vi "Joystick Outputs.vi"(0 "JoystickDevRef":T1) -> (1 "Buttons":T4, 2 "Axis":T3, 3 "POV":cluster{"POV":i16})   [LabVIEW 2020]
uses:
  <vilib>/Rock Robotics/WPI/Joystick/WPI_JoystickDevRef.ctl
  <vilib>/Rock Robotics/WPI/Joystick/WPI_JoystickDeviceEnum.ctl
panel:
  out "POV BL":bool
  out "POV BR":bool
  out "POV TR":bool
  out "POV TR":bool
  out "POV B":bool
  out "POV T":bool
  out "POV L":bool
  out "POV R":bool
  out "POV C":bool
  out "\"x' 13":bool
  out "\"x' 12":bool
  out "\"x' 11":bool
  out "\"x' 10":bool
  out "\"x' 9":bool
  out "\"x' 8":bool
  out "\"x' 7":bool
  out "\"x' 2":bool
  out "\"x' 6":bool
  out "\"x' 4":bool
  out "\"x' 3":bool
  out "\"x' 2":bool
  out "\"x'":bool
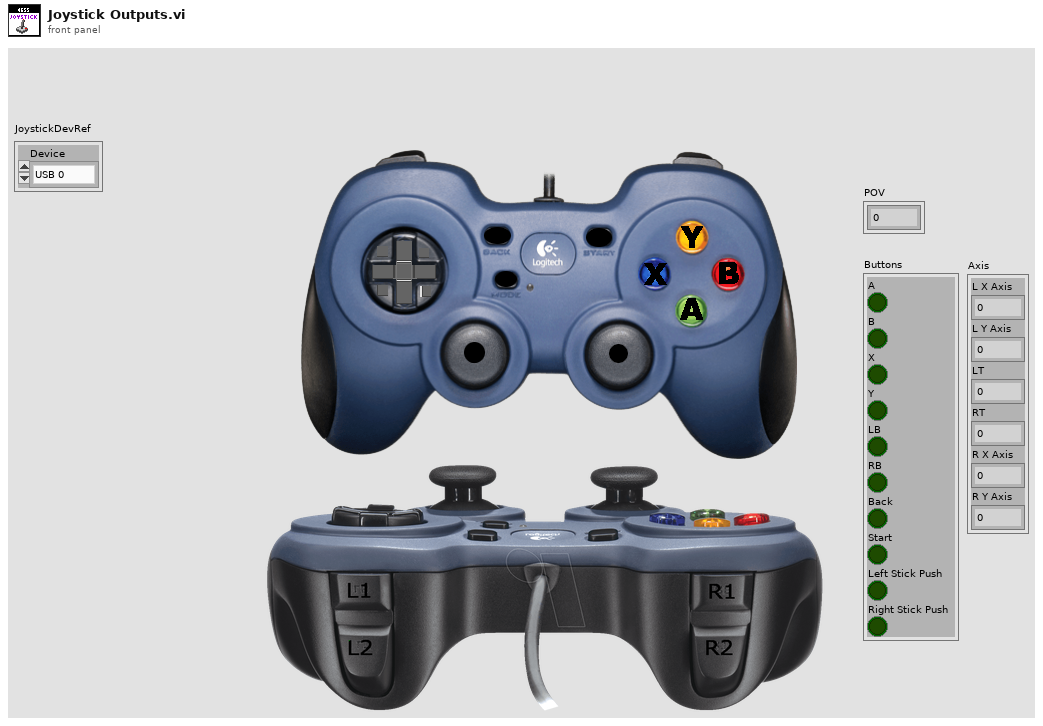
[diagram p1: front panel]
types:
  T1 = typedef "WPI_JoystickDevRef.ctl" = cluster{"Device":T2}
  T2 = typedef "WPI_JoystickDeviceEnum.ctl" = enum16{"USB 0", "USB 1", "USB 2", "USB 3", "USB 4", "USB 5"}
  T3 = cluster{"L X Axis":dbl, "L Y Axis":dbl, "LT":dbl, "RT":dbl, "R X Axis":dbl, "R Y Axis":dbl}
  T4 = cluster{"A":bool, "B":bool, "X":bool, "Y":bool, "LB":bool, "RB":bool, "Back":bool, "Start":bool, "Left Stick Push":bool, "Right Stick Push":bool}
  T5 = cluster{"Buttons[0]":bool, "Buttons[1]":bool, "Buttons[2]":bool, "Buttons[3]":bool, "Buttons[4]":bool, "Buttons[5]":bool, "Buttons[6]":bool, "Buttons[7]":bool, "Buttons[8]":bool, "Buttons[9]":bool}
  T6 = cluster{"Axes[0]":dbl, "Axes[1]":dbl, "Axes[2]":dbl, "Axes[3]":dbl, "Axes[4]":dbl, "Axes[5]":dbl}
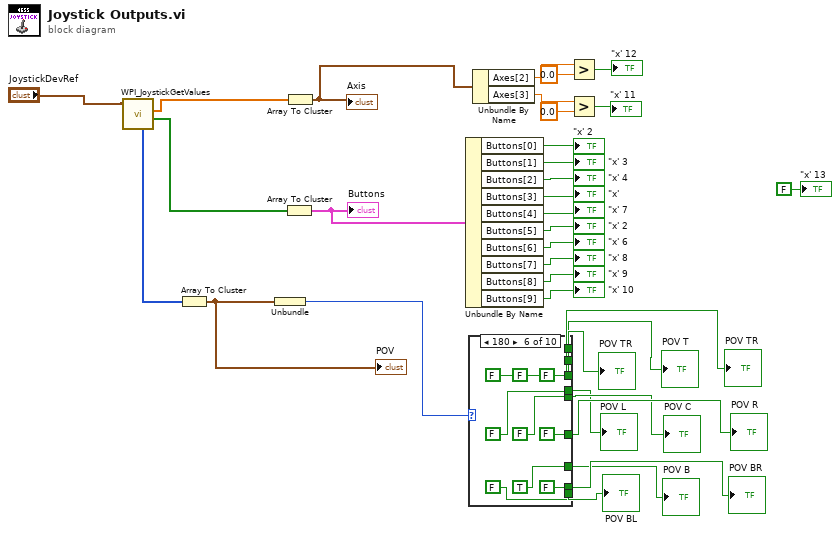
[diagram p0: block diagram]
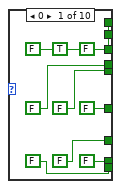
[diagram p2: hidden frame]
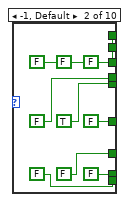
[diagram p3: hidden frame]
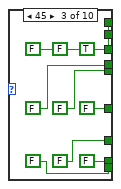
[diagram p4: hidden frame]
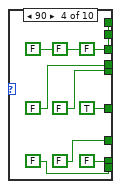
[diagram p5: hidden frame]
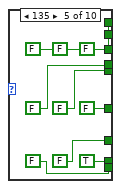
[diagram p6: hidden frame]
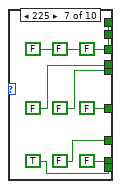
[diagram p7: hidden frame]
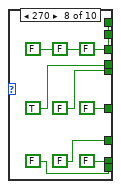
[diagram p8: hidden frame]
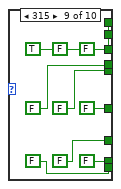
[diagram p9: hidden frame]
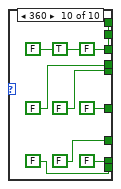
[diagram p10: hidden frame]
diagram:
  n1 = call <vilib>:"WPI_JoystickGetValues.vi"("JoystickDevRef"="JoystickDevRef") -> ("Buttons"=w34:bool[], "Axes"=w33:dbl[], "POVs"=w32:i16[])  [unwired: 6 in, 2 out]
  n2 = Array To Cluster(array=w32) -> (cluster=w14:cluster{"POVs[0]":i16})
  "POV" <- w14
  n3 = Unbundle(w14) -> ("POVs[0]"=w3:i16)
  n4 = Array To Cluster(array=w34) -> (cluster=w31:T5)
  "Buttons" <- w31
  n5 = Array To Cluster(array=w33) -> (cluster=w20:T6)
  "Axis" <- w20
  n6 = Unbundle By Name(w31) -> ("Buttons[0]"=→"\"x' 2":bool, "Buttons[1]"=→"\"x' 3":bool, "Buttons[2]"=→"\"x' 4":bool, "Buttons[3]"=→"\"x'":bool, "Buttons[4]"=→"\"x' 7":bool, "Buttons[5]"=→"\"x' 2":bool, "Buttons[6]"=→"\"x' 6":bool, "Buttons[7]"=→"\"x' 8":bool, "Buttons[8]"=→"\"x' 9":bool, "Buttons[9]"=→"\"x' 10":bool)
  n7 = case shown="180" w3 {
    tunnel: [FALSE ("POV TR") FALSE ("POV TR") FALSE ("POV TR") FALSE ("POV TR") FALSE ("POV TR") FALSE ("POV TR") FALSE ("POV TR") FALSE ("POV TR") TRUE ("POV TR") FALSE ("POV TR")] -> w12
    tunnel: [TRUE ("POV T") FALSE ("POV T") FALSE ("POV T") FALSE ("POV T") FALSE ("POV T") FALSE ("POV T") FALSE ("POV T") FALSE ("POV T") FALSE ("POV T") TRUE ("POV T")] -> w11
    tunnel: [FALSE ("POV TR") FALSE ("POV TR") TRUE ("POV TR") FALSE ("POV TR") FALSE ("POV TR") FALSE ("POV TR") FALSE ("POV TR") FALSE ("POV TR") FALSE ("POV TR") FALSE ("POV TR")] -> w10
    tunnel: [FALSE ("POV TR") FALSE ("POV TR") FALSE ("POV TR") TRUE ("POV TR") FALSE ("POV TR") FALSE ("POV TR") FALSE ("POV TR") FALSE ("POV TR") FALSE ("POV TR") FALSE ("POV TR")] -> w9
    tunnel: [FALSE ("POV T") TRUE ("POV T") FALSE ("POV T") FALSE ("POV T") FALSE ("POV T") FALSE ("POV T") FALSE ("POV T") FALSE ("POV T") FALSE ("POV T") FALSE ("POV T")] -> w8
    tunnel: [FALSE ("POV TR") FALSE ("POV TR") FALSE ("POV TR") FALSE ("POV TR") FALSE ("POV TR") FALSE ("POV TR") FALSE ("POV TR") TRUE ("POV TR") FALSE ("POV TR") FALSE ("POV TR")] -> w7
    tunnel: [FALSE ("POV TR") FALSE ("POV TR") FALSE ("POV TR") FALSE ("POV TR") TRUE ("POV TR") FALSE ("POV TR") FALSE ("POV TR") FALSE ("POV TR") FALSE ("POV TR") FALSE ("POV TR")] -> w6
    tunnel: [FALSE ("POV T") FALSE ("POV T") FALSE ("POV T") FALSE ("POV T") FALSE ("POV T") TRUE ("POV T") FALSE ("POV T") FALSE ("POV T") FALSE ("POV T") FALSE ("POV T")] -> w5
    tunnel: [FALSE ("POV TR") FALSE ("POV TR") FALSE ("POV TR") FALSE ("POV TR") FALSE ("POV TR") FALSE ("POV TR") TRUE ("POV TR") FALSE ("POV TR") FALSE ("POV TR") FALSE ("POV TR")] -> w4
    frame 0 {
    }
    frame -1, Default {
    }
    frame 45 {
    }
    frame 90 {
    }
    frame 135 {
    }
    frame 180 {
    }
    frame 225 {
    }
    frame 270 {
    }
    frame 315 {
    }
    frame 360 {
    }
  }
  "POV C" <- w8
  "POV R" <- w9
  "POV L" <- w7
  "POV T" <- w11
  "POV B" <- w5
  "POV TR" <- w10
  "POV TR" <- w12
  "POV BR" <- w6
  "POV BL" <- w4
  n8 = Unbundle By Name(w20) -> ("Axes[2]"=w19:dbl, "Axes[3]"=w18:dbl)
  n9 = Greater?(x=w19, y=0.0) -> (0:→"\"x' 12":bool)
  n10 = Greater?(x=w18, y=0.0) -> (0:→"\"x' 11":bool)
  "\"x' 13" <- FALSE ("\"x' 13")
